vi "Directory Parsing.vi"() -> ()   [LabVIEW 2020]
panel:
  out "stripped path":path
  out "Current VI's Path (+ Relative)":path
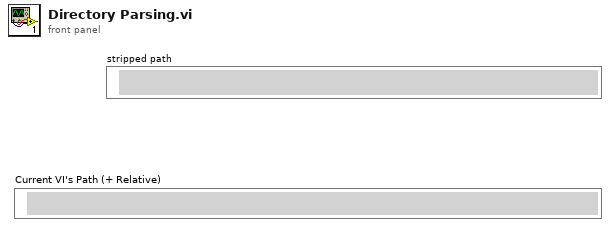
[diagram p1: front panel]
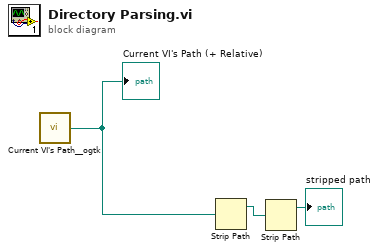
[diagram p0: block diagram]
diagram:
  n1 = call <userlib>:"Current VI's Path__ogtk.vi"() -> ("Current VI's Path (+ Relative)"=w3:path)  [unwired: 1 in]
  "Current VI's Path (+ Relative)" <- w3
  n2 = Strip Path(path=w3) -> (stripped path=w2:path)  [unwired: 1 out]
  n3 = Strip Path(path=w2) -> (stripped path=→"stripped path":path)  [unwired: 1 out]
